vi "CMO_Query.vi"(0 "System no.":i32=1 min=1 max=4 step=1, 2 "Axes to query":string[](array[string]), 3 "All axes?":bool, 4 "Axis identifier?":bool=TRUE, 5 "error in":errorcluster) -> (14 "Control mode":dbl[](array[numeric]) format="%.6f", 19 "error out":errorcluster)   [LabVIEW 2020]
doc: "Returns the current control mode. \n\nC-413: If All axes? = TRUE, then Axis identifier? can be FALSE"
panel:
  # "Returns the current control mode."
  # "If all axes: use"
  # "Query"
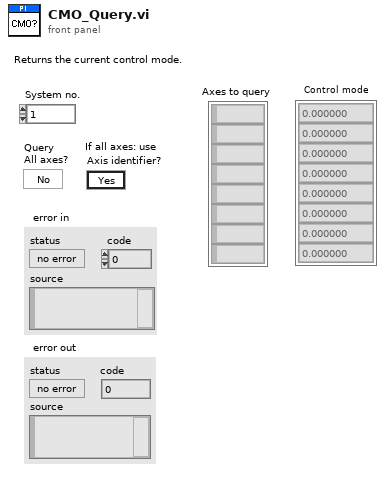
[diagram p1: front panel]
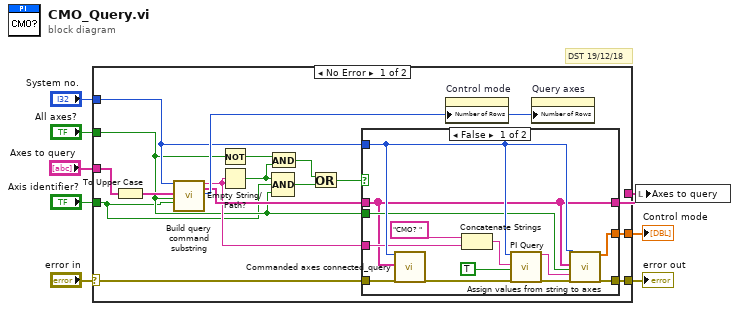
[diagram p0: block diagram]
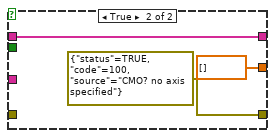
[diagram p2: hidden frame]
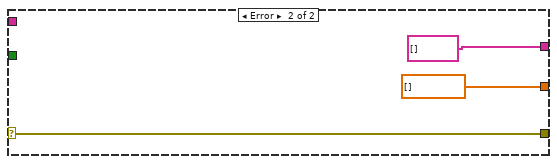
[diagram p3: hidden frame]
diagram:
  # "DST 19/12/18"
  n1 = case shown="No Error" "error in" {
    selector: "error in" -> [w15 w42]
    tunnel: [w25 dbl[] [] ("Values")] -> w8
    tunnel: "Axes to query" -> [w24 _]
    tunnel: [w16 w42] -> w6
    tunnel: "System no." -> [w21 _]
    tunnel: [w9 string[] [] ("Axes to query out")] -> w4
    tunnel: "Axis identifier?" -> [w10 _]
    tunnel: "All axes?" -> [w11 _]
    frame No Error {
      n2 = To Upper Case(1:w24) -> (0:w23:string[])
      n3 = call "Build query command substring.vi"("System no."=w21, "Axes to query in"=w23, "Query\nAll axes?"=w11, "For all axes: use\nAxis identifier?"=w10) -> ("Command substring"=w14:string, "Axes to query out"=w20:string[], "Number of rows"=w22:u32)  [unwired: 2 in, 11 out]
      n4 = Not(x=w11) -> (.not. x?=w19:bool)
      n5 = Empty String/Path?(string/path=w14) -> (empty?=w13:bool)
      n6 = And(x=w19, y=w13) -> (x .and. y?=w18:bool)
      n7 = Compound Arithmetic op=AND(w13, w10, w11) -> (w17:bool)
      n8 = Or(x=w18, y=w17) -> (x .or. y?=w12:bool)
      n9 = case shown="False" w12 {
        tunnel: [w35 dbl[] [] ("Values")] -> w25
        tunnel: w21 -> [w34 _]
        tunnel: w20 -> [w26 w39]
        tunnel: w11 -> [w33 _]
        tunnel: [w31 errorcluster {"status"=TRUE, "code"=100, "source"="CMO? no axis specified"} ("error out")] -> w16
        tunnel: w15 -> [w30 _]
        tunnel: w14 -> [w27 _]
        tunnel: [w26 w39] -> w9
        frame False {
          n10 = call "Commanded axes connected_query.vi"("System no."=w34, "Commanded axes"=w26, "error in"=w30) -> ("error out"=w32:errorcluster)  [unwired: 1 in, 15 out]
          n11 = Concatenate Strings("CMO? ", w27) -> (w36:string)
          n12 = call "PI Query.vi"("System no."=w34, "String to send"=w36, "Attach termination char.?"=TRUE ("Attach Linefeed?"), "error in"=w32) -> ("String read"=w29:string, "error out"=w28:errorcluster)  [unwired: 3 in, 11 out]
          n13 = call "Assign values from string to axes.vi"("System no."=w34, "Queried axes"=w26, "All axes queried?"=w33, "Input String"=w29, "error in"=w28) -> ("Values"=w35:dbl[], "error out"=w31:errorcluster)  [unwired: 4 in, 9 out]
        }
        frame True {
        }
      }
      n14 = property on="Control mode" class="Arr (strict)"("Number of Rows"=w22) -> ()  [unwired: 2 in, 2 out]
      n15 = property on="Query axes" class="Arr (strict)"("Number of Rows"=w22) -> ()  [unwired: 2 in, 2 out]
    }
    frame Error {
    }
  }
  "error out" <- w6
  "Control mode" <- w8
  n16 = local write "Axes to query"(w4) -> ()
